vi "23384_Davis_Poku_Amankwa_Amankwa.DavisPoku.MNE1201.1.1_348251_1095259683.vi"() -> ()   [LabVIEW 2018]
panel:
  out "Integer?":bool
  in  "Number":dbl
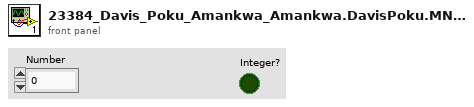
[diagram p1: front panel]
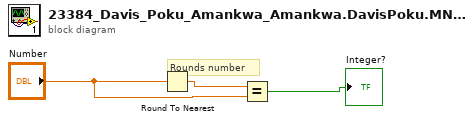
[diagram p0: block diagram]
diagram:
  # "Rounds number"
  n1 = Round To Nearest(number="Number") -> (nearest integer value=w3:dbl)
  n2 = Equal?(x=w3, y="Number") -> (x = y?=→"Integer?":bool)
